vi "Initialize.vi"(8 "error in (no error)":errorcluster, 9 "Reset (True)":bool, 10 "ID Query (True)":bool, 11 "VISA resource name":refnum<visa-resource-name>="PG-AT") -> (0 "error out":errorcluster, 3 "VISA resource name out":refnum<visa-resource-name>="PG-AT")   [LabVIEW 2019, in "Pulse Rider PG-1000.lvlib"]
doc: "Establishes communication with the instrument and optionally performs an instrument identification query and/or an instrument reset. It also places the instrument in a default state needed for other instrument driver operations. Therefore, call this VI before calling other instrument driver VIs for this instrument. Generally, you need to call the Initialize VI only once at the beginning of an application."
uses:
  <instrlib>/LV_PulseRiderPG1000/Pulse Rider PG-1000.lvlib
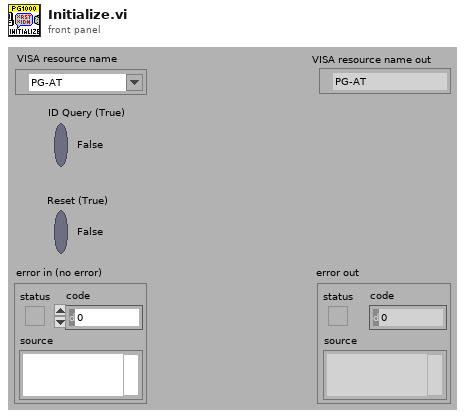
[diagram p1: front panel]
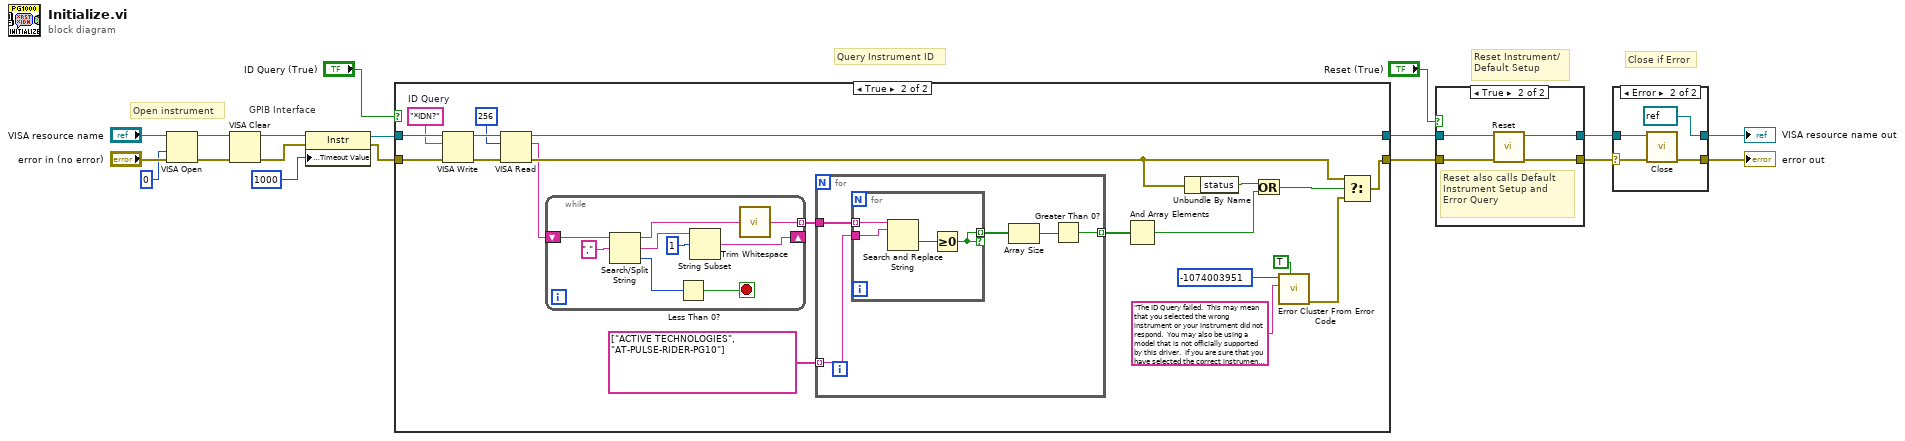
[diagram p0: block diagram]
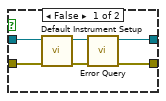
[diagram p3: hidden frame]
diagram:
  # "GPIB Interface"
  # "Close if Error"
  # "Query Instrument ID"
  # "Reset Instrument/\nDefault Setup"
  # "Open instrument"
  n1 = VISA Open(access mode=u32 0, error in (no error)="error in (no error)", VISA resource name="VISA resource name") -> (VISA resource name=w8:refnum<visa-resource-name>, error out=w7:errorcluster)  [unwired: 2 in]
  n2 = VISA Clear(VISA resource name=w8, error in (no error)=w7) -> (VISA resource name out=w6:refnum<visa-resource-name>, error out=w5:errorcluster)
  n3 = property class="Instr"(reference=w6, error in=w5, "General Settings:Timeout Value"=u32 1000) -> (reference out=w11:refnum<visa-resource-name>, error out=w10:errorcluster)
  n4 = case shown="True" "ID Query (True)" {
    tunnel: [w19 w40] -> w17
    tunnel: [w20 w37] -> w18
    tunnel: w11 -> [w20 w38]
    tunnel: w10 -> [w19 w39]
    frame False {
    }
    frame True {
      w33 = "*IDN?"  # ID Query
      n5 = VISA Write(VISA resource name=w38, write buffer=w33, error in (no error)=w39) -> (VISA resource name out=w36:refnum<visa-resource-name>, error out=w35:errorcluster)  [unwired: 1 out]
      n6 = VISA Read(VISA resource name=w36, byte count=u32 256, error in (no error)=w35) -> (VISA resource name out=w37:refnum<visa-resource-name>, read buffer=w22:string, error out=w28:errorcluster)  [unwired: 1 out]
      n7 = while {
        shift-right: [w44] -> _
        shift-left: w22 -> [w47]
        tunnel: [w42] -> w25 mode=indexing
        stop <- w45 stop-if-true
        n8 = Search/Split String(string=w47, search string/char (-)=",") -> (substring before match=w41:string, match + rest of string=w43:string, offset of match=w46:i32)  [unwired: 1 in]
        n9 = Less Than 0?(x=w46) -> (x < 0?=w45:bool)
        n10 = String Subset(string=w43, offset (0)=1) -> (substring=w44:string)  [unwired: 1 in]
        n11 = call <vilib>:"Trim Whitespace.vi"("string"=w41) -> ("trimmed string"=w42:string)  [unwired: 1 in]
      }
      n12 = for {
        tunnel: w25 -> [w54]
        tunnel: string[] ["ACTIVE TECHNOLOGIES", "AT-PULSE-RIDER-PG10"] -> [w53] mode=indexing
        tunnel: [w50] -> w23 mode=indexing
        n13 = for {
          tunnel: w54 -> [w57] mode=indexing
          tunnel: w53 -> [w58]
          tunnel: [w56] -> w52 mode=indexing if=w56
          n14 = Search and Replace String(input string=w57, search string=w58) -> (offset past replacement=w55:i32)  [unwired: 6 in, 3 out]
          n15 = Greater Or Equal To 0?(x=w55) -> (x >= 0?=w56:bool)
        }
        n16 = Array Size(array=w52) -> (size(s)=w51:i32)
        n17 = Greater Than 0?(x=w51) -> (x > 0?=w50:bool)
      }
      n18 = And Array Elements(Boolean array=w23) -> (logical AND=w21:bool)
      n19 = Unbundle By Name(w28) -> ("status"=w27:bool)
      n20 = Or(x=w27, y=w21) -> (x .or. y?=w26:bool)
      n21 = call <vilib>:"Error Cluster From Error Code.vi"("show call chain? (False)"=TRUE, "error message (\"\")"="The ID Query failed.  This may mean that you selected the wrong instrument or your instrument did not respond.  You may also be using a model that is not officially supported by this driver.  If you are sure that you have selected the correct instrument and it is responding, try disabling the ID Query." ("Source (VI Name)"), "error code (0)"=-1074003951 ("Code")) -> ("error out"=w32:errorcluster)  [unwired: 6 in]
      n22 = Select(t=w28, s=w26, f=w32) -> (s? t:f=w40:errorcluster)
    }
  }
  n23 = case shown="True" "Reset (True)" {
    tunnel: w17 -> [w63 w65]
    tunnel: [w60 w68] -> w1
    tunnel: w18 -> [w64 w66]
    tunnel: [w61 w67] -> w2
    frame False {
      n24 = call <instrlib>:"Default Instrument Setup.vi"("error in (no error)"=w63, "VISA resource name"=w64) -> ("error out"=w59:errorcluster, "VISA resource name out"=w62:refnum<visa-resource-name>)  [unwired: 8 in]
      n25 = call <instrlib>:"Error Query.vi"("error in (no error)"=w59, "VISA resource name"=w62) -> ("error out"=w60:errorcluster, "VISA resource name out"=w61:refnum<visa-resource-name>)  [unwired: 6 in, 2 out]
    }
    frame True {
      # "Reset also calls Default Instrument Setup and Error Query"
      n26 = call <instrlib>:"Reset.vi"("error in (no error)"=w65, "VISA resource name"=w66) -> ("error out"=w68:errorcluster, "VISA resource name out"=w67:refnum<visa-resource-name>)  [unwired: 8 in]
    }
  }
  n27 = case shown="Error" w1 {
    selector: w1 -> [w69 w72]
    tunnel: w2 -> [w70 w73]
    tunnel: [w70 refnum<visa-resource-name> refnum ("VISA resource name out")] -> w4
    tunnel: [w69 w74] -> w3
    frame No Error {
    }
    frame Error {
      n28 = call <instrlib>:"Close.vi"("error in (no error)"=w72, "VISA resource name"=w73) -> ("error out"=w74:errorcluster)  [unwired: 9 in]
    }
  }
  "VISA resource name out" <- w4
  "error out" <- w3
